vi "Control_Get Attributes.vi"(8 "error in (no error)":errorcluster, 10 "Only Get DVR":bool, 11 "Control In":refnum<class "Control.lvclass">) -> (0 "error out":errorcluster, 1 "DataRef":refnum<data-value>, 2 "Data":T1, 3 "Control Out":refnum<class "Control.lvclass">)   [LabVIEW 2015, in "Front Panel Publisher.lvlib" / "Control.lvclass"]
uses:
  Control.lvclass
  Attributes.ctl
  Text_class/Text.lvclass
  Control.lvclass/Control.ctl
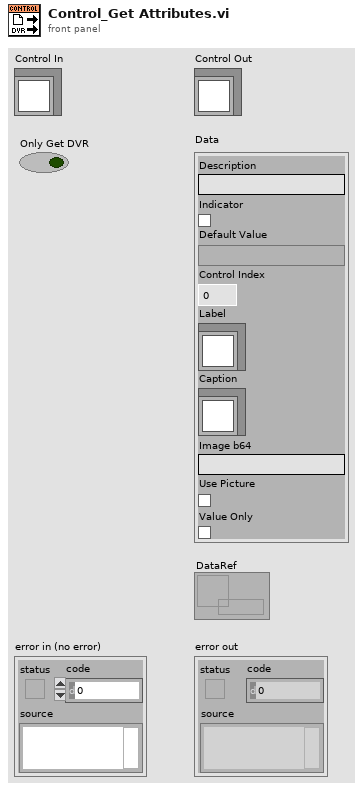
[diagram p1: front panel]
types:
  T1 = typedef "Front Panel Publisher.lvlib/Control.lvclass/Attributes.ctl" = cluster{"Description":string, "Indicator":bool, "Default Value":variant, "Control Index":i32, "Label":refnum<class "Text.lvclass">, "Caption":refnum<class "Text.lvclass">, "Image b64":string, "Use Picture":bool, "Value Only":bool}
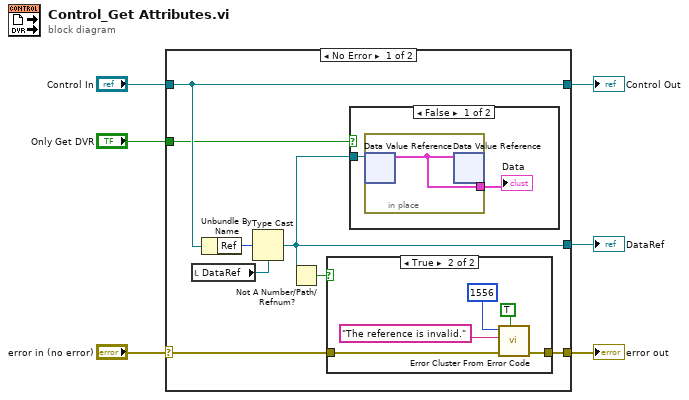
[diagram p0: block diagram]
diagram:
  n1 = case shown="No Error" "error in (no error)" {
    selector: "error in (no error)" -> [w8 w24]
    tunnel: [w7 w24] -> w5
    tunnel: [w14 w25] -> w3
    tunnel: "Control In" -> [w14 w25]
    tunnel: [w10 _] -> w2
    tunnel: "Only Get DVR" -> [w11 _]
    frame No Error {
      n2 = local read "DataRef"() -> (w12:refnum<data-value>)
      n3 = Unbundle By Name(w14) -> ("Ref"=w13:u32)
      n4 = Type Cast(type=w12, x=w13) -> (*(type *) &x=w10:refnum<data-value>)
      n5 = Not A Number/Path/Refnum?(number/path/refnum=w10) -> (NaN/Path/Refnum?=w9:bool)
      n6 = case shown="True" w9 {
        tunnel: w8 -> [w15 w17]
        tunnel: [w15 w16] -> w7
        frame False {
        }
        frame True {
          n7 = call <vilib>:"Error Cluster From Error Code.vi"("show call chain? (False)"=TRUE, "error in (no error)"=w17, "error message (\"\")"="The reference is invalid." ("source"), "error code (0)"=1556 ("code")) -> ("error out"=w16:errorcluster)  [unwired: 5 in]
        }
      }
      n8 = case shown="False" w11 {
        tunnel: w10 -> [w22 _]
        frame False {
          n9 = in-place {
            in-place-border: [w23] -> w21
            n10 = in-place-dvr #1(w22) -> (w23:T1)  [unwired: 1 out]
            n11 = in-place-dvr #1(w23) -> ()  [unwired: 2 out]
          }
          "Data" <- w21
        }
        frame True {
        }
      }
    }
    frame Error {
    }
  }
  "error out" <- w5
  "Control Out" <- w3
  "DataRef" <- w2
